vi "PH_Beckhoff_StepMot.set GUI Elements to Default.vi"(0 "i ref in":refnum<vi>, 5 "error in":errorcluster) -> (14 "i ref out":refnum<vi>, 19 "error out":errorcluster)   [LabVIEW 2014, in "PH_Beckhoff_StepMot.lvlib"]
doc: "Within this VI captions are set and GUI elements which are not in use are set not to be visible."
uses:
  PH_Beckhoff_StepMot.lvlib
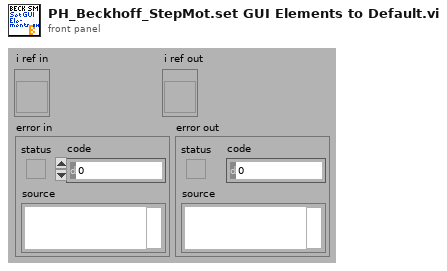
[diagram p1: front panel]
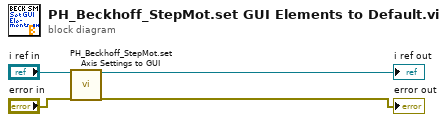
[diagram p0: block diagram]
diagram:
  n1 = call "PH_Beckhoff_StepMot.set Axis Settings to GUI.vi"("VI in"="i ref in", "error in (no error)"="error in") -> ("VI out"=→"i ref out":refnum<vi>, "error out"=→"error out":errorcluster)  [unwired: 16 in]
